vi "FixedCurrentAging.vi"(0 "VSet (V)":sgl, 1 "Device Code":i32=21, 2 "ID":i32=1, 3 "Channel":u8(ring) items=["1", "2", "3", "4", "5", "6", "7", "8", "9", "10", "11", "12", "13", "14", "15", "16"], 4 "instance":i32, 5 "JV after\nevery (min)":dbl=15.0 caption="Time Target (s)", 7 "Record_every_dT":sgl=1.0, 8 "device area (cm2)":dbl=0.16 caption="Time Target (s)", 11 "error in (no error)":errorcluster, 12 "start time":timestamp, 14 "AgingFile":path=path "C:/EC-Lab Development Package/Examples/Labview/V12/DefaultAging") -> (15 "error out":errorcluster)   [LabVIEW 2020]
uses:
  base_xml.llb/Type Descriptor Enumeration__ogtk.ctl
  ActiveArray.vi
  <vilib>/Utility/file.llb/Write Delimited Spreadsheet (DBL).vi
  IntensityTemperature.vi
panel:
  in  "CP Parameters":T1={"Steps"=[{"vs_initial"=FALSE, "Current_step"=0.0, "Duration_step"=1.0}, {"vs_initial"=FALSE, "Current_step"=0.0001, "Duration_step"=3.0}, {"vs_initial"=FALSE, "Current_step"=0.005, "Duration_step"=10.0}], "Step_number"=1, "N_Cycles"=0, "Record_every_dE"=0.5, "Record_every_dT"=0.05, "I_Range"=8, "E_Range"=3, "Bandwidth"=5, "em"=1, "ce"=0, "tb"=0.0001} {"tb" min=2.5e-05 max=1 format="%^_3e"; "ce" items=["Standard", "CE to ground"]; "N_Cycles" min=0 max=1000000; "Step_number" min=0 max=99; "E_Range" items=["±2.5V", "±5V", "±10V", "Auto"]; "Bandwidth" items=["1"=1, "2"=2, "3"=3, "4"=4, "5"=5, "6"=6, "7"=7, "8"=8, "9"=9]; "Record_every_dT" min=0.0001 max=1000 format="%^_3e"; "Record_every_dE" format="%^_3e"; "I_Range" items=["1pA", "1nA", "10nA", "100nA", "1µA", "10µA", "100µA", "1mA", "10mA", "100mA", "1A", "Booster"]; "Steps"."Duration_step" min=0.001 max=80000 format="%^_3e"; "Steps"."Current_step" min=-150 max=150 format="%^_3e"}
  out "finished":bool
  out "XY Graph 2":cluster{"Data 101":sgl[], "Data 101":dbl[]}(graph) caption="XY Graph"
  out "Number\nof points":i32=255
  in  "Current measurement":enum16{"P(t)", "Ewe(t)", "I(t)"}(ring) caption="Draw"
  out "time (s)":sgl
  out "V (V)":sgl
  out "J (mA/cm2)":sgl
  out "P (mW/cm2)":sgl
  out "Aging Data":sgl[][](array[numeric])
  in  "stop 4":bool
  out "CAData":sgl[][](array[numeric])=[[0.0, -0.00011507986, 2.9229916e-06, 1.0], [0.010008001, -0.00048330438, 2.9229916e-06, 1.0], [0.020016002, -0.00048330438, 2.9229916e-06, 1.0], [0.030024001, -0.0007121685, 6.7342776e-06, 1.0], [0.040032003, -0.0007121685, 3.6852487e-06, 1.0], [0.050040003, -0.00063588045, 6.362202e-07, 1.0], [0.060048003, -0.00048330438, 5.2097635e-06, 1.0], [0.070056, -0.0004070163, 2.1607345e-06, 1.0], [0.080064006, -0.00017815214, 3.6852487e-06, 1.0], [0.090072006, -0.0004070163, 3.6852487e-06, 1.0], [0.100080006, -0.0004070163, 2.1607345e-06, 1.0], [0.110088006, -0.00063588045, 2.9229916e-06, 1.0], [0.120096005, -0.0005595924, 2.9229916e-06, 1.0], [0.130104, -0.0007121685, 5.2097635e-06, 1.0], [0.140112, -0.00033072825, 5.2097635e-06, 1.0], [0.15012, -0.00063588045, 2.9229916e-06, 1.0], [0.16012801, -0.0007884566, 1.3984774e-06, 1.0], [0.170136, -0.0004070163, 5.2097635e-06, 1.0], [0.18014401, -0.00063588045, 3.6852487e-06, 1.0], [0.190152, -0.00063588045, 5.97202e-06, 1.0], [0.20016001, -0.0007121685, 5.2097635e-06, 1.0], [0.210168, -0.00033072825, 2.9229916e-06, 1.0], [0.22017601, -0.0007121685, 1.3984774e-06, 1.0], [0.230184, -0.00063588045, 5.97202e-06, 1.0], [0.24019201, -0.0007884566, 5.97202e-06, 1.0], [0.2502, -0.00063588045, 4.447506e-06, 1.0], [0.260208, -0.00063588045, 4.447506e-06, 1.0], [0.27021602, -0.0007884566, 3.6852487e-06, 1.0], [0.280224, -0.00025444018, 2.9229916e-06, 1.0], [0.290232, -0.00063588045, 4.447506e-06, 1.0], [0.30024, -0.0007884566, 5.2097635e-06, 1.0], [0.31024802, -0.00048330438, 2.9229916e-06, 1.0], [0.32025602, -0.00063588045, 2.1607345e-06, 1.0], [0.330264, -0.00063588045, 3.6852487e-06, 1.0], [0.340272, -0.00063588045, 2.9229916e-06, 1.0], [0.35028002, -0.00017815214, 5.2097635e-06, 1.0], [0.36028802, -0.0007884566, 5.97202e-06, 1.0], [0.370296, -0.00063588045, 2.9229916e-06, 1.0], [0.380304, -0.00086474465, 6.7342776e-06, 1.0], [0.39031202, -0.0004070163, 2.9229916e-06, 1.0], [0.40032002, -0.0007884566, 6.362202e-07, 1.0], [0.410328, -0.0007121685, 2.1607345e-06, 1.0], [0.420336, -0.0007884566, 6.7342776e-06, 1.0], [0.43034402, -0.00063588045, 1.3984774e-06, 1.0], [0.44035202, -0.00063588045, 2.9229916e-06, 1.0], [0.45036003, -0.00063588045, 2.1607345e-06, 1.0], [0.460368, -0.00048330438, 4.447506e-06, 1.0], [0.470376, -0.00048330438, 4.447506e-06, 1.0], [0.48038402, -0.0004070163, 2.9229916e-06, 1.0], [0.49039203, -0.00033072825, 5.2097635e-06, 1.0], [0.5004, -0.00048330438, 5.2097635e-06, 1.0], [0.51040804, -0.0005595924, 5.2097635e-06, 1.0], [0.520416, -0.0005595924, 5.97202e-06, 1.0], [0.530424, -0.0007121685, 5.2097635e-06, 1.0], [0.54043204, -0.0004070163, 2.9229916e-06, 1.0], [0.55044, -0.00025444018, 5.2097635e-06, 1.0], [0.560448, -0.00048330438, 2.9229916e-06, 1.0], [0.570456, -0.0004070163, 4.447506e-06, 1.0], [0.580464, -0.0004070163, 2.9229916e-06, 1.0], [0.59047204, -0.00063588045, 2.1607345e-06, 1.0], [0.60048, -0.0007884566, 2.1607345e-06, 1.0], [0.610488, -0.00048330438, 5.2097635e-06, 1.0], [0.62049603, -0.0004070163, 2.9229916e-06, 1.0], [0.630504, -0.0007884566, 3.6852487e-06, 1.0], [0.64051205, -0.0007884566, 2.9229916e-06, 1.0], [0.65052, -0.0005595924, 5.97202e-06, 1.0], [0.660528, -0.00048330438, 2.9229916e-06, 1.0], [0.67053604, -0.00063588045, 4.447506e-06, 1.0], [0.680544, -0.00086474465, 4.447506e-06, 1.0], [0.690552, -0.00063588045, 3.6852487e-06, 1.0], [0.70056003, -0.00063588045, 1.3984774e-06, 1.0], [0.710568, -0.0005595924, 4.447506e-06, 1.0], [0.72057605, -0.00048330438, 2.9229916e-06, 1.0], [0.730584, -0.00048330438, 3.6852487e-06, 1.0], [0.740592, -0.0007884566, 4.447506e-06, 1.0], [0.75060004, -0.0005595924, 3.6852487e-06, 1.0], [0.760608, -0.0005595924, 2.9229916e-06, 1.0], [0.77061605, -0.0007884566, 4.447506e-06, 1.0], [0.78062403, -0.0010173208, 2.1607345e-06, 1.0], [0.790632, -0.00063588045, 2.1607345e-06, 1.0], [0.80064005, -0.00025444018, 2.9229916e-06, 1.0], [0.810648, -0.0005595924, 3.6852487e-06, 1.0], [0.820656, -0.00017815214, 3.6852487e-06, 1.0], [0.83066404, -0.0005595924, 4.447506e-06, 1.0], [0.840672, -0.0005595924, 1.3984774e-06, 1.0], [0.85068005, -0.00063588045, 5.2097635e-06, 1.0], [0.86068803, -0.0007884566, 5.97202e-06, 1.0], [0.870696, -0.0004070163, 4.447506e-06, 1.0], [0.88070405, -0.00033072825, 4.447506e-06, 1.0], [0.890712, -0.0005595924, 3.6852487e-06, 1.0], [0.90072006, -0.0005595924, 4.447506e-06, 1.0], [0.91072804, -0.0007121685, 4.447506e-06, 1.0], [0.920736, -0.00063588045, 2.1607345e-06, 1.0], [0.93074405, -0.0005595924, 5.2097635e-06, 1.0], [0.940752, -0.0004070163, 2.1607345e-06, 1.0], [0.95076, -0.0004070163, 2.1607345e-06, 1.0], [0.96076804, -0.00025444018, 2.9229916e-06, 1.0], [0.970776, -0.00063588045, 3.6852487e-06, 1.0], [0.98078406, -0.00063588045, 2.9229916e-06, 1.0], [0.99079204, 0.0001270001, 2.1607345e-06, 1.0], [1.0008, 0.09945406, 5.5518736e-05, 1.0], [1.010808, 0.09960663, 2.3503935e-05, 1.0], [1.0208161, 0.09945406, 2.2741679e-05, 1.0], [1.0308241, 0.099759206, 2.5790707e-05, 1.0], [1.040832, 0.09930148, 2.4266194e-05, 1.0], [1.05084, 0.099377766, 2.1217164e-05, 1.0], [1.060848, 0.09945406, 2.2741679e-05, 1.0], [1.0708561, 0.09953035, 2.1217164e-05, 1.0], [1.0808641, 0.09953035, 2.3503935e-05, 1.0], [1.090872, 0.09953035, 2.3503935e-05, 1.0], [1.10088, 0.09968292, 2.4266194e-05, 1.0], [1.110888, 0.09945406, 2.4266194e-05, 1.0], [1.120896, 0.09953035, 2.6552963e-05, 1.0], [1.1309041, 0.099377766, 2.6552963e-05, 1.0], [1.140912, 0.09953035, 2.502845e-05, 1.0], [1.15092, 0.09922519, 2.1217164e-05, 1.0], [1.160928, 0.09953035, 2.3503935e-05, 1.0], [1.170936, 0.099377766, 1.969265e-05, 1.0], [1.1809441, 0.09930148, 2.4266194e-05, 1.0], [1.1909521, 0.09953035, 2.4266194e-05, 1.0], [1.20096, 0.09953035, 2.3503935e-05, 1.0], [1.210968, 0.09953035, 2.4266194e-05, 1.0], [1.220976, 0.09968292, 2.2741679e-05, 1.0], [1.2309841, 0.09960663, 2.4266194e-05, 1.0], [1.2409921, 0.0998355, 2.4266194e-05, 1.0], [1.251, 0.09945406, 2.1217164e-05, 1.0], [1.261008, 0.09968292, 2.502845e-05, 1.0], [1.271016, 0.09930148, 2.4266194e-05, 1.0], [1.2810241, 0.09968292, 1.8930392e-05, 1.0], [1.2910321, 0.09930148, 2.4266194e-05, 1.0], [1.30104, 0.09930148, 2.5790707e-05, 1.0], [1.311048, 0.09907261, 2.4266194e-05, 1.0], [1.321056, 0.09945406, 2.1217164e-05, 1.0], [1.3310641, 0.09968292, 2.5790707e-05, 1.0], [1.3410721, 0.09914891, 2.1979422e-05, 1.0], [1.3510801, 0.09945406, 2.502845e-05, 1.0], [1.361088, 0.09945406, 2.5790707e-05, 1.0], [1.371096, 0.09960663, 2.1217164e-05, 1.0], [1.381104, 0.09930148, 2.4266194e-05, 1.0], [1.3911121, 0.09930148, 2.4266194e-05, 1.0], [1.4011201, 0.09998807, 2.4266194e-05, 1.0], [1.411128, 0.09968292, 2.4266194e-05, 1.0], [1.421136, 0.09960663, 2.1217164e-05, 1.0], [1.431144, 0.09998807, 2.3503935e-05, 1.0], [1.4411521, 0.09968292, 2.1217164e-05, 1.0], [1.4511601, 0.09953035, 2.5790707e-05, 1.0], [1.461168, 0.09960663, 2.5790707e-05, 1.0], [1.471176, 0.09968292, 2.2741679e-05, 1.0], [1.481184, 0.09930148, 2.4266194e-05, 1.0], [1.4911921, 0.09945406, 2.2741679e-05, 1.0], [1.5012001, 0.09960663, 2.0454907e-05, 1.0], [1.511208, 0.09945406, 2.3503935e-05, 1.0], [1.521216, 0.099377766, 1.969265e-05, 1.0], [1.531224, 0.09930148, 2.1217164e-05, 1.0], [1.5412321, 0.09914891, 2.2741679e-05, 1.0], [1.5512401, 0.09953035, 2.2741679e-05, 1.0], [1.5612481, 0.099377766, 2.2741679e-05, 1.0], [1.571256, 0.099377766, 2.5790707e-05, 1.0], [1.581264, 0.099759206, 2.4266194e-05, 1.0], [1.5912721, 0.09968292, 2.2741679e-05, 1.0], [1.6012801, 0.09930148, 2.4266194e-05, 1.0], [1.6112881, 0.09930148, 2.4266194e-05, 1.0], [1.621296, 0.09960663, 2.1217164e-05, 1.0], [1.631304, 0.09968292, 2.5790707e-05, 1.0], [1.641312, 0.09953035, 2.5790707e-05, 1.0], [1.6513201, 0.09930148, 2.502845e-05, 1.0], [1.6613281, 0.09945406, 2.4266194e-05, 1.0], [1.671336, 0.09953035, 2.1217164e-05, 1.0], [1.681344, 0.099377766, 2.4266194e-05, 1.0], [1.691352, 0.09960663, 2.2741679e-05, 1.0], [1.7013601, 0.09968292, 2.3503935e-05, 1.0], [1.7113681, 0.09907261, 2.5790707e-05, 1.0], [1.7213761, 0.09953035, 2.4266194e-05, 1.0], [1.731384, 0.099377766, 2.2741679e-05, 1.0], [1.741392, 0.09960663, 2.502845e-05, 1.0], [1.7514001, 0.09953035, 2.502845e-05, 1.0], [1.7614081, 0.09945406, 2.6552963e-05, 1.0], [1.7714161, 0.099377766, 2.502845e-05, 1.0], [1.781424, 0.09960663, 2.5790707e-05, 1.0], [1.791432, 0.09907261, 2.502845e-05, 1.0], [1.8014401, 0.09930148, 2.0454907e-05, 1.0], [1.8114481, 0.09968292, 2.1979422e-05, 1.0], [1.8214561, 0.09930148, 2.2741679e-05, 1.0], [1.831464, 0.09930148, 2.4266194e-05, 1.0], [1.841472, 0.09914891, 2.0454907e-05, 1.0], [1.85148, 0.099377766, 2.2741679e-05, 1.0], [1.8614881, 0.09953035, 2.502845e-05, 1.0], [1.8714961, 0.09945406, 2.3503935e-05, 1.0], [1.881504, 0.09907261, 2.502845e-05, 1.0], [1.891512, 0.099377766, 2.2741679e-05, 1.0], [1.90152, 0.09945406, 2.5790707e-05, 1.0], [1.9115281, 0.09953035, 2.5790707e-05, 1.0], [1.9215361, 0.099759206, 2.4266194e-05, 1.0], [1.9315441, 0.09945406, 2.6552963e-05, 1.0], [1.941552, 0.09945406, 2.0454907e-05, 1.0], [1.95156, 0.09945406, 2.5790707e-05, 1.0], [1.9615681, 0.09991179, 2.5790707e-05, 1.0], [1.9715761, 0.09945406, 2.3503935e-05, 1.0], [1.9815841, 0.09930148, 2.3503935e-05, 1.0], [1.991592, 0.09960663, 2.5790707e-05, 1.0], [2.0016, 0.19969657, 6.3903564e-05, 1.0], [2.0116081, 0.19939142, 4.256037e-05, 1.0], [2.021616, 0.19931513, 4.408488e-05, 1.0], [2.031624, 0.1994677, 4.332262e-05, 1.0], [2.0416322, 0.199544, 4.332262e-05, 1.0], [2.05164, 0.1994677, 4.4847136e-05, 1.0], [2.0616481, 0.19962028, 4.332262e-05, 1.0], [2.071656, 0.19977286, 4.332262e-05, 1.0], [2.081664, 0.19992544, 4.256037e-05, 1.0], [2.0916722, 0.19977286, 4.4847136e-05, 1.0], [2.10168, 0.19977286, 4.408488e-05, 1.0], [2.1116881, 0.20007801, 4.4847136e-05, 1.0], [2.121696, 0.19992544, 4.103585e-05, 1.0], [2.131704, 0.199544, 4.256037e-05, 1.0], [2.1417122, 0.199544, 4.6371653e-05, 1.0], [2.15172, 0.19969657, 4.256037e-05, 1.0], [2.1617281, 0.199544, 4.256037e-05, 1.0], [2.171736, 0.19984914, 4.256037e-05, 1.0], [2.181744, 0.1994677, 4.256037e-05, 1.0], [2.1917522, 0.20000172, 4.256037e-05, 1.0], [2.20176, 0.199544, 4.6371653e-05, 1.0], [2.2117682, 0.1994677, 4.0273593e-05, 1.0], [2.221776, 0.19969657, 4.332262e-05, 1.0], [2.231784, 0.19962028, 4.332262e-05, 1.0], [2.241792, 0.199544, 4.408488e-05, 1.0], [2.2518, 0.19977286, 4.332262e-05, 1.0], [2.2618082, 0.1994677, 4.408488e-05, 1.0], [2.271816, 0.19969657, 4.6371653e-05, 1.0], [2.281824, 0.19969657, 4.408488e-05, 1.0], [2.291832, 0.1994677, 4.332262e-05, 1.0], [2.30184, 0.19984914, 4.408488e-05, 1.0], [2.3118482, 0.19923884, 3.9511335e-05, 1.0], [2.321856, 0.19962028, 4.256037e-05, 1.0], [2.331864, 0.19969657, 4.1798106e-05, 1.0], [2.341872, 0.19969657, 4.6371653e-05, 1.0], [2.35188, 0.19969657, 4.4847136e-05, 1.0], [2.3618882, 0.19969657, 4.6371653e-05, 1.0], [2.371896, 0.19939142, 4.103585e-05, 1.0], [2.3819041, 0.19939142, 4.332262e-05, 1.0], [2.391912, 0.1994677, 4.103585e-05, 1.0], [2.40192, 0.19962028, 4.1798106e-05, 1.0], [2.4119282, 0.19962028, 4.4847136e-05, 1.0], [2.421936, 0.1994677, 4.332262e-05, 1.0], [2.4319441, 0.19977286, 4.408488e-05, 1.0], [2.441952, 0.20007801, 4.408488e-05, 1.0], [2.45196, 0.19984914, 4.5609395e-05, 1.0], [2.4619682, 0.19962028, 4.256037e-05, 1.0], [2.471976, 0.19984914, 4.4847136e-05, 1.0], [2.4819841, 0.19939142, 4.6371653e-05, 1.0], [2.491992, 0.199544, 4.1798106e-05, 1.0], [2.502, 0.19984914, 4.408488e-05, 1.0], [2.5120082, 0.19931513, 4.332262e-05, 1.0], [2.522016, 0.199544, 4.6371653e-05, 1.0], [2.5320241, 0.199544, 4.4847136e-05, 1.0], [2.542032, 0.19931513, 4.408488e-05, 1.0]] format="%.2f"
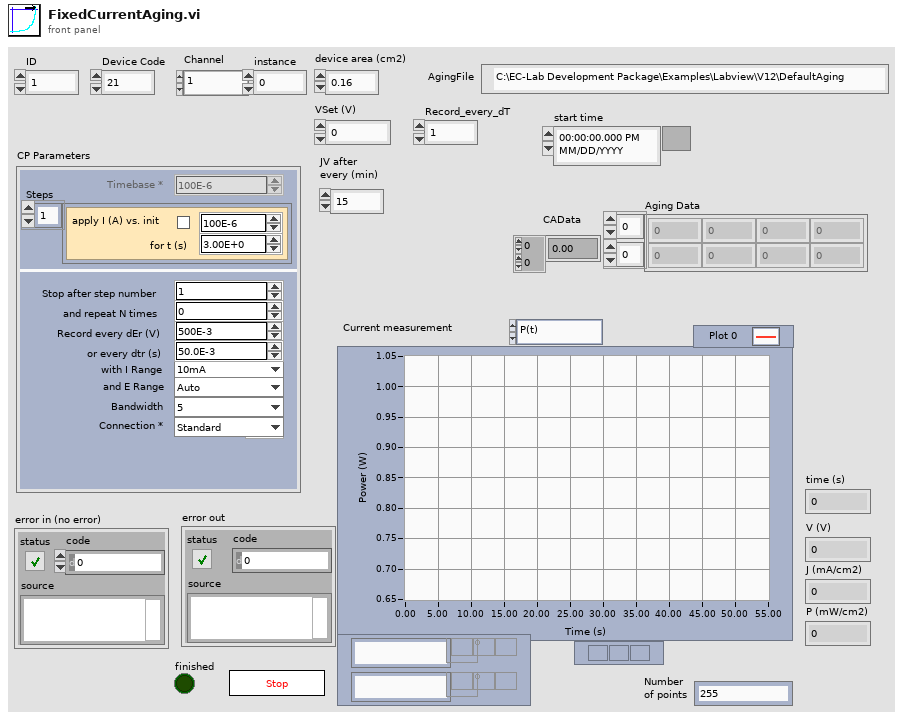
[diagram p1: front panel]
types:
  T1 = cluster{"Steps":cluster{"vs_initial":bool, "Current_step":sgl, "Duration_step":sgl}[], "Step_number":i32, "N_Cycles":i32, "Record_every_dE":sgl, "Record_every_dT":sgl, "I_Range":u16, "E_Range":u16, "Bandwidth":u16, "em":u16, "ce":u16, "tb":sgl}
  T2 = typedef "Type Descriptor Enumeration__ogtk.ctl" = enum8{"<Null>", "I8", "I16", "I32", "I64", "U8", "U16", "U32", "U64", "SGL", "DBL", "EXT", "CSG", "CDB", "CXT", "0x0F", "0x10", "0x11", "0x12", "0x13", "0x14", "Enum U8", "Enum U16", "Enum U32", "Enum U64", "SGL PQ", "DBL PQ", "EXT PQ", "CSG PQ", "CDB PQ", "CXT PQ", "0x1F", "0x20", "Boolean", "0x22", "0x23", "0x24", "0x25", "0x26", "0x27", "0x28", "0x29", "0x2A", "0x2B", "0x2C", "0x2D", "0x2E", "0x2F", "String", "0x31", "Path", "Pict", "0x34", "0x35", "0x36", "DAQ", "0x38", "0x39", "0x3A", "0x3B", "0x3C", "0x3D", "0x3E", "0x3F", "Array", "0x41", "0x42", "0x43", "0x44", "0x45", "0x46", "0x47", "0x48", "0x49", "0x4A", "0x4B", "0x4C", "0x4D", "0x4E", "0x4F", "Cluster", "0x51", "0x52", "Variant", "Waveform", "0x55", "0x56", "0x57", "0x58", "0x59", "0x5A", "0x5B", "0x5C", "0x5D", "0x5E", "0x5F", "0x60", "0x61", "0x62", "0x63", "0x64", "0x65", "0x66", "0x67", "0x68", "0x69", "0x6A", "0x6B", "0x6C", "0x6D", "0x6E", "0x6F", "Refnum"}
  T3 = cluster{"Data Type":T2, "Format String":string}[]
  T4 = cluster{"vs_initial":bool, "Current_step":sgl, "Duration_step":sgl}[]
  T5 = cluster{"vs_initial":bool, "Current_step":sgl, "Duration_step":sgl}
  T6 = cluster{"Label":string, "type":i32, "valeur":u32, "index":i32}[]
  T7 = cluster{"IRQskipped":i32, "NbRaws":i32, "NbCols":i32, "Technique Index":i32, "TechniqueID":i32, "PrcessIndex":i32, "loop":i32, "StartTime":dbl, "MuxPad":i32}
  T8 = cluster{"State":i32, "MemFilled":i32, "TimeBase":sgl, " Ewe":sgl, " EweRangeMin":sgl, " EweRangeMax":sgl, "Ece":sgl, "EceRangeMin":sgl, "EceRangeMax":sgl, "Eoverflow":i32, "I":sgl, "IRange":i32, "Ioverflow":i32, "ElapsedTime":sgl, "Freq":sgl, "Rcomp":sgl, "Saturation":sgl, "OptErr":i32, "OptPos":i32}
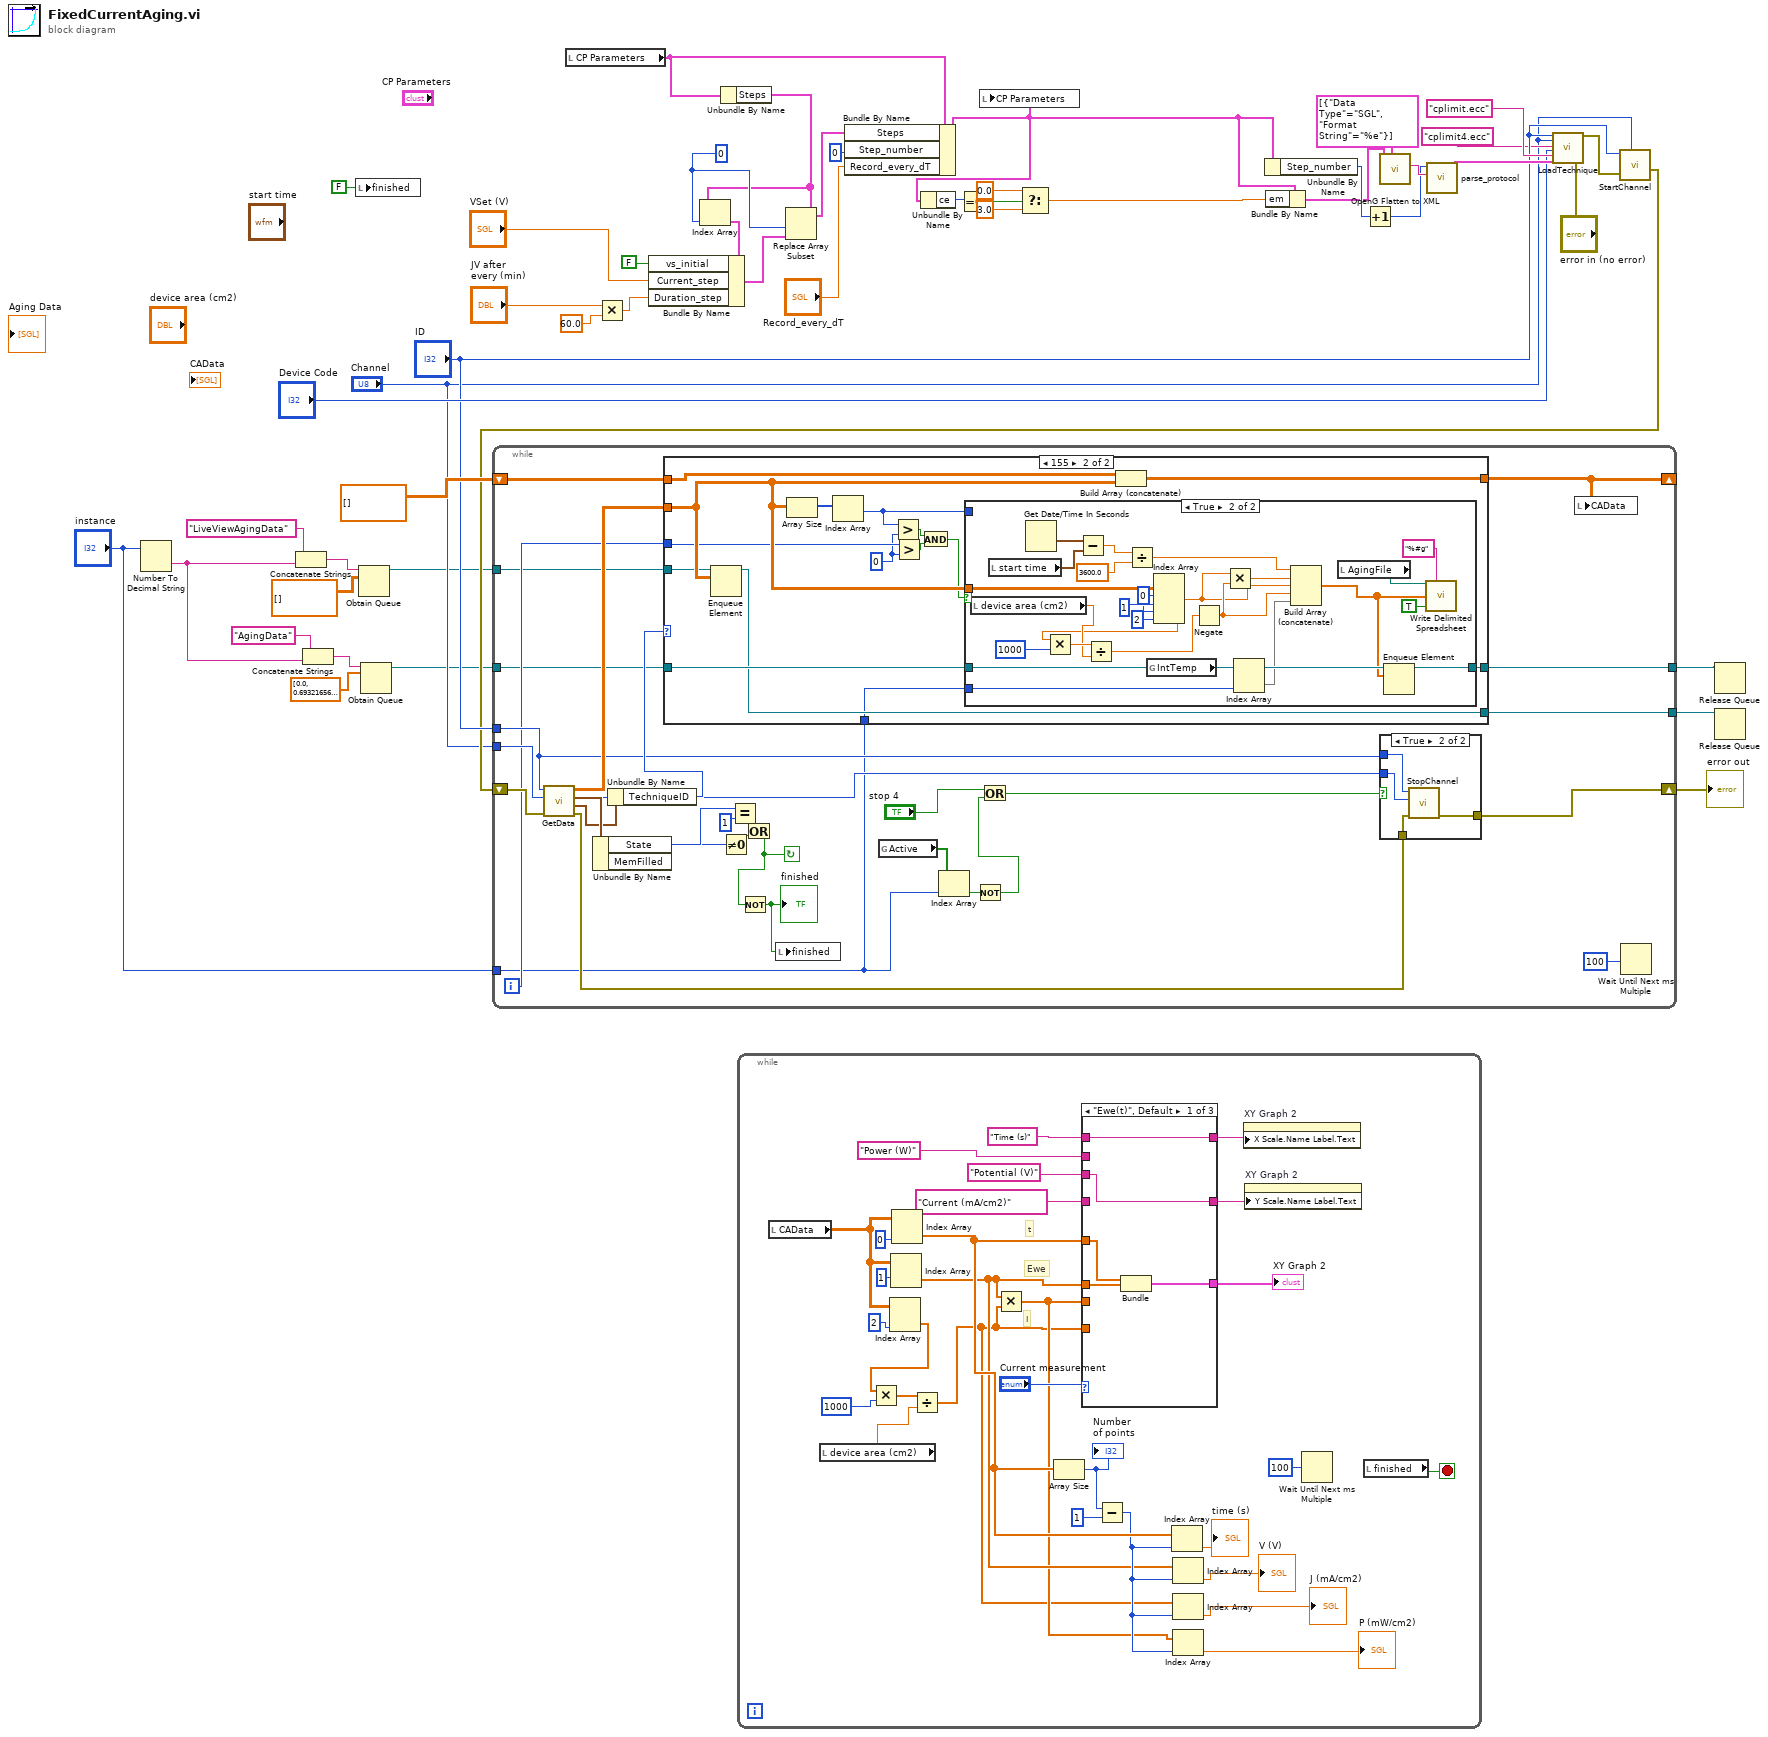
[diagram p0: block diagram]
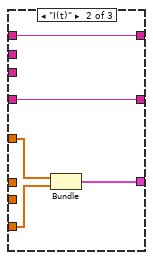
[diagram p2: hidden frame]
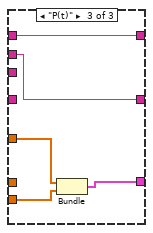
[diagram p3: hidden frame]
diagram:
  w35 = 0 ("index")
  n1 = Number To Decimal String(number="instance") -> (decimal integer string=w6:string)  [unwired: 1 in]
  n2 = Concatenate Strings("LiveViewAgingData" ("name (unnamed)"), w6) -> (w12:string)
  n3 = Concatenate Strings("AgingData" ("name (unnamed)"), w6) -> (w8:string)
  n4 = local write "finished"(FALSE ("finished")) -> ()
  n5 = Obtain Queue(name (unnamed)=w12, element data type=sgl[][] []) -> (queue out=w5:refnum<queue>)  [unwired: 3 in, 2 out]
  n6 = Obtain Queue(name (unnamed)=w8, element data type=dbl[] [0.0, 0.6932165634222212, 0.002936372303467471, 0.2869923716049554, 0.0005841850023007069, 0.39914193749427795, 0.001463602161096093, 0.0, 0.0, 0.0, 0.0, 0.0, 0.0, inf] ("appended array 2")) -> (queue out=w4:refnum<queue>)  [unwired: 3 in, 2 out]
  n7 = local read "CP Parameters"() -> (w31:T1)
  n8 = Multiply(x="JV after\nevery (min)", y=60.0) -> (x*y=w29:dbl)
  n9 = Unbundle By Name(w31) -> ("Steps"=w34:T4)
  n10 = Index Array(array=w34, index=w35) -> (element=w33:T5)
  n11 = Bundle By Name(cluster=w33, "vs_initial"=FALSE, "Current_step"="VSet (V)", "Duration_step"=w29) -> (w36:T5)
  n12 = while {
    stop <- w76 stop-if-true
    # "I"
    # "Ewe"
    # "t"
    n13 = local read "CAData"() -> (w66:sgl[][])
    n14 = local read "device area (cm2)"() -> (w52:dbl)
    n15 = Index Array(array=w66, index (col)=2 ("indice désactivé (col)")) -> (element=w50:sgl[])  [unwired: 1 in]
    n16 = Multiply(x=w50, y=1000) -> (x*y=w53:sgl[])
    n17 = Index Array(array=w66, index (col)=1 ("Index")) -> (element=w59:sgl[])  [unwired: 1 in]
    n18 = Index Array(array=w66, index (col)=0 ("Index")) -> (element=w61:sgl[])  [unwired: 1 in]
    n19 = Divide(x=w53, y=w52) -> (x/y=w49:dbl[])
    n20 = Multiply(x=w59, y=w49) -> (x*y=w58:dbl[])
    n21 = Array Size(array=w61) -> (size(s)=w63:i32)
    "Number\nof points" <- w63
    n22 = case shown="\"Ewe(t)\", Default" "Current measurement" {
      tunnel: w61 -> [w82 w83 w90]
      tunnel: [w79 w84 w88] -> w65
      tunnel: "Potential (V)" ("Y Scale.Name Label.Text") -> [w81 _ _]
      tunnel: "Current (mA/cm2)" ("Y Scale.Name Label.Text") -> [_ w87 _]
      tunnel: [w81 w87 w91] -> w70
      tunnel: [w80 w86 w92] -> w69
      tunnel: "Time (s)" ("Y Scale.Name Label.Text") -> [w80 w86 w92]
      tunnel: w59 -> [w78 _ _]
      tunnel: w49 -> [_ w85 _]
      tunnel: "Power (W)" ("Y Scale.Name Label.Text") -> [_ _ w91]
      tunnel: w58 -> [_ _ w89]
      frame "Ewe(t)", Default {
        n23 = Bundle("CAData"=w82, "CAData"=w78) -> (w79:cluster{"CAData":sgl[], "CAData":sgl[]})  [unwired: 1 in]
      }
      frame "I(t)" {
        n24 = Bundle("CAData"=w83, w85) -> (w84:cluster{"CAData":sgl[], dbl[]})  [unwired: 1 in]
      }
      frame "P(t)" {
        n25 = Bundle("CAData"=w90, w89) -> (w88:cluster{"CAData":sgl[], dbl[]})  [unwired: 1 in]
      }
    }
    "XY Graph 2" <- w65
    n26 = Subtract(x=w63, y=1) -> (x-y=w60:i32)
    n27 = Index Array(array=w61, index=w60) -> (element=→"time (s)":sgl)
    n28 = Index Array(array=w59, index=w60) -> (element=→"V (V)":sgl)
    n29 = Index Array(array=w49, index=w60) -> (element=→"J (mA/cm2)":dbl)
    n30 = Index Array(array=w58, index=w60) -> (element=→"P (mW/cm2)":dbl)
    n31 = property on="XY Graph 2" class="XYGraph (strict)"("X Scale.Name Label.Text"=w69) -> ()  [unwired: 2 in, 2 out]
    n32 = property on="XY Graph 2" class="XYGraph (strict)"("Y Scale.Name Label.Text"=w70) -> ()  [unwired: 2 in, 2 out]
    n33 = Wait Until Next ms Multiple(millisecond multiple=u32 100) -> ()  [unwired: 1 out]
    n34 = local read "finished"() -> (w76:bool)
  }
  n35 = Replace Array Subset(array=w34, new element=w36, index=w35) -> (w30:T4)
  n36 = Bundle By Name(cluster=w31, "Steps"=w30, "Step_number"=0, "Record_every_dT"="Record_every_dT") -> (w27:T1)
  n37 = Unbundle By Name(w27) -> ("ce"=w39:u16)
  n38 = Equal To 0?(x=w39) -> (x = 0?=w38:bool)
  n39 = local write "CP Parameters"(w27) -> ()
  n40 = Select(t=0.0, s=w38, f=3.0) -> (s? t:f=w42:dbl)
  n41 = Unbundle By Name(w27) -> ("Step_number"=w44:i32)
  n42 = Bundle By Name(cluster=w27, "em"=w42) -> (w37:T1)
  n43 = Increment(x=w44) -> (x+1=w43:i32)
  n44 = call "OpenG Flatten to XML.vi"("Type Formats (default)"=T3 [{"Data Type"=enum."SGL", "Format String"="%e"}] ("Type Formats"), "LabVIEW Data"=w37) -> ("XML String"=w47:string)  [unwired: 8 in, 1 out]
  n45 = call "parse_protocol.vi"("XML String In"=w47, "index array"=w43) -> ("Params Values"=w46:T6)  [unwired: 7 in]
  n46 = call "LoadTechnique.vi"("ID"="ID", "Selected Channel"="Channel", "FName4"="cplimit4.ecc" ("FName"), "Device Code"="Device Code", "FName"="cplimit.ecc", "Protocol Parameters"=w46, "error in (no error)"="error in (no error)") -> ("error out"=w48:errorcluster)  [unwired: 12 in]
  n47 = call "StartChannel.vi"("error in (no error)"=w48, "Channel"="Channel", "ID"="ID") -> ("error out"=w20:errorcluster)  [unwired: 8 in]
  n48 = while {
    shift-right: [w117] -> w18
    shift-left: w20 -> [w119]
    shift-right: [w100] -> _
    shift-left: sgl[][] [] -> [w115]
    tunnel: "Channel" -> [w99]
    tunnel: "ID" -> [w109]
    tunnel: w5 -> [w97]
    tunnel: w4 -> [w96]
    tunnel: [w95] -> w3
    tunnel: [w94] -> w2
    tunnel: "instance" -> [w93]
    i -> [w98]
    stop <- w108 continue-if-true
    n49 = call "GetData.vi"("error in (no error)"=w119, "Channel"=w99, "ID"=w109) -> ("error out"=w106:errorcluster, "Data information"=w111:T7, "Current values"=w114:T8, "Data"=w116:dbl[][])  [unwired: 5 in]
    n50 = Unbundle By Name(w114) -> ("State"=w113:i32, "MemFilled"=w112:i32)
    n51 = Unbundle By Name(w111) -> ("TechniqueID"=w110:i32)
    n52 = case shown="155" w110 {
      tunnel: w116 -> [_ w143]
      tunnel: w115 -> [w130 w145]
      tunnel: [w130 w144] -> w100
      tunnel: w98 -> [_ w141]
      tunnel: w97 -> [w128 w135]
      tunnel: w96 -> [w129 w134]
      tunnel: [w129 w133] -> w95
      tunnel: [w128 w132] -> w94
      tunnel: w93 -> [_ w131]
      frame 0, Default {
      }
      frame 155 {
        w139 = 0 ("y")
        n53 = Enqueue Element(queue=w135, element=w143) -> (queue out=w132:refnum<queue>)  [unwired: 2 in, 2 out]
        n54 = Array Size(array=w143) -> (size(s)=w142:i32[])
        n55 = Index Array(array=w142) -> (element=w140:i32)  [unwired: 1 in]
        n56 = Greater?(x=w140, y=w139) -> (0:w137:bool)
        n57 = Greater?(x=w141, y=w139) -> (0:w138:bool)
        n58 = And(x=w137, y=w138) -> (x .and. y?=w136:bool)
        n59 = case shown="True" w136 {
          tunnel: w143 -> [_ w160]
          tunnel: w140 -> [_ _]
          tunnel: w134 -> [w146 w154]
          tunnel: [w146 w153] -> w133
          tunnel: w131 -> [_ w150]
          frame False {
          }
          frame True {
            w149 = 0 ("disabled index (row)")
            n60 = local read "device area (cm2)"() -> (w157:dbl)
            n61 = local read "start time"() -> (w166:timestamp)
            n62 = Get Date/Time In Seconds() -> (seconds since 1Jan1904=w167:timestamp)
            n63 = Subtract(x=w167, y=w166) -> (x-y=w169:dbl)
            n64 = Divide(x=w169, y=3600.0) -> (x/y=w148:dbl)
            n65 = global read "IntensityTemperature.vi" "IntTemp"() -> (w152:dbl[][])
            n66 = Index Array(array=w160, index (row) #1=w149, index (col) #1=1 ("Index"), index (row) #2=w149, index (col) #2=2 ("index (col)")) -> (element #1=w161:dbl, element #2=w156:dbl)
            n67 = Multiply(x=w156, y=1000) -> (x*y=w159:dbl)
            n68 = Divide(x=w159, y=w157) -> (x/y=w155:dbl)
            n69 = Negate(x=w155) -> (-x=w162:dbl)
            n70 = Multiply(x=w161, y=w162) -> (x*y=w163:dbl)
            n71 = Index Array(array=w152, index (col)=w150) -> (element=w151:dbl[])  [unwired: 1 in]
            n72 = Build Array (concatenate)(w148, w163, w161, w162, w151) -> (w147:dbl[])
            n73 = local read "AgingFile"() -> (w171:path)
            n74 = Enqueue Element(queue=w154, element=w147) -> (queue out=w153:refnum<queue>)  [unwired: 2 in, 2 out]
            n75 = call-poly <vilib>:"Write Delimited Spreadsheet.vi"("file path (dialog if empty)"=w171, "format (%.3f)"="%#g", "1D data"=w147, "append to file? (new file:F)"=TRUE ("append to file? (F)")) -> ()  [unwired: 10 in, 2 out]
          }
        }
        n76 = Build Array (concatenate)(w145, w143) -> (w144:dbl[][])
      }
    }
    n77 = Not Equal To 0?(x=w112) -> (x != 0?=w120:bool)
    n78 = Equal?(x=w113, y=1) -> (x = y?=w121:bool)
    n79 = Or(x=w121, y=w120) -> (x .or. y?=w108:bool)
    n80 = Not(x=w108) -> (.not. x?=w107:bool)
    "finished" <- w107
    n81 = local write "finished"(w107) -> ()
    n82 = global read "ActiveArray.vi" "Active"() -> (w105:bool[])
    n83 = Index Array(array=w105, index=w93) -> (element=w104:bool)
    n84 = Not(x=w104) -> (.not. x?=w103:bool)
    n85 = Or(x="stop 4", y=w103) -> (x .or. y?=w102:bool)
    n86 = case shown="True" w102 {
      tunnel: [w123 w125] -> w117
      tunnel: w99 -> [_ w127]
      tunnel: w109 -> [_ w126]
      tunnel: w106 -> [w123 w124]
      frame False {
      }
      frame True {
        n87 = call "StopChannel.vi"("error in (no error)"=w124, "Channel"=w127, "ID"=w126) -> ("error out"=w125:errorcluster)  [unwired: 8 in]
      }
    }
    n88 = local write "CAData"(w100) -> ()
    n89 = Wait Until Next ms Multiple(millisecond multiple=u32 100) -> ()  [unwired: 1 out]
  }
  "error out" <- w18
  n90 = Release Queue(queue=w3) -> ()  [unwired: 2 in, 3 out]
  n91 = Release Queue(queue=w2) -> ()  [unwired: 2 in, 3 out]
